vi "TraverseDoAllChannels.vi"(0 "Current Pulses positions for all channels":sgl[](array[numeric]), 1 "Current Pos In Eng units of all channels":sgl[](array[numeric]) format="%.2f", 2 "Counters Reset?":bool, 5 "Backlash Compensation?":bool, 7 "Home":T3, 9 "Mode":T4, 11 "Position Steps":sgl[][](array[numeric]) format="%.2f", 12 "Channel Properties":T1[](array[typedef]) {"Current Pos" format="%.2f"; "Backlash/Eng units" format="%.2f"; "Pulses/rev" format="%.2f"; "Pos Tolerance" format="%.2f"; "Pulses/unit" format="%.2f"; "Acc. Min" format="%.2f"; "Acc. Max" format="%.2f"; "Vel. Min" format="%.2f"; "Vel. Max" format="%.2f"; "Acc. Default" format="%.2f"; "Vel. Default" format="%.2f"}, 13 "Last Part of Move?":bool, 14 "Traverse Name":string="EnFlo Tunnel") -> (4 "Achieved Pos In Eng units of all channels":sgl[](array[numeric]) format="%.2f", 6 "Current Pulses positions for all channels Out":sgl[](array[numeric]), 8 "Moved?":bool, 10 "Error String":string, 15 "Channel Properties Out":T1[](array[typedef]) {"Current Pos" format="%.2f"; "Backlash/Eng units" format="%.2f"; "Pulses/rev" format="%.2f"; "Pos Tolerance" format="%.2f"; "Pulses/unit" format="%.2f"; "Acc. Min" format="%.2f"; "Acc. Max" format="%.2f"; "Vel. Min" format="%.2f"; "Vel. Max" format="%.2f"; "Acc. Default" format="%.2f"; "Vel. Default" format="%.2f"})   [LabVIEW 2022 SP3]
uses:
  Anemometry/Anemometry Sub Vis/Gen Trav/Trav_mode.ctl
  Anemometry/Anemometry Sub Vis/Controls/Home.ctl
  ~subVIs/DriveProperties.ctl
  ~subVIs/Traverse Type.ctl
  ~subVIs/DriveGotoCluster.ctl
  ~subVIs/DriveConfigGlobal.vi
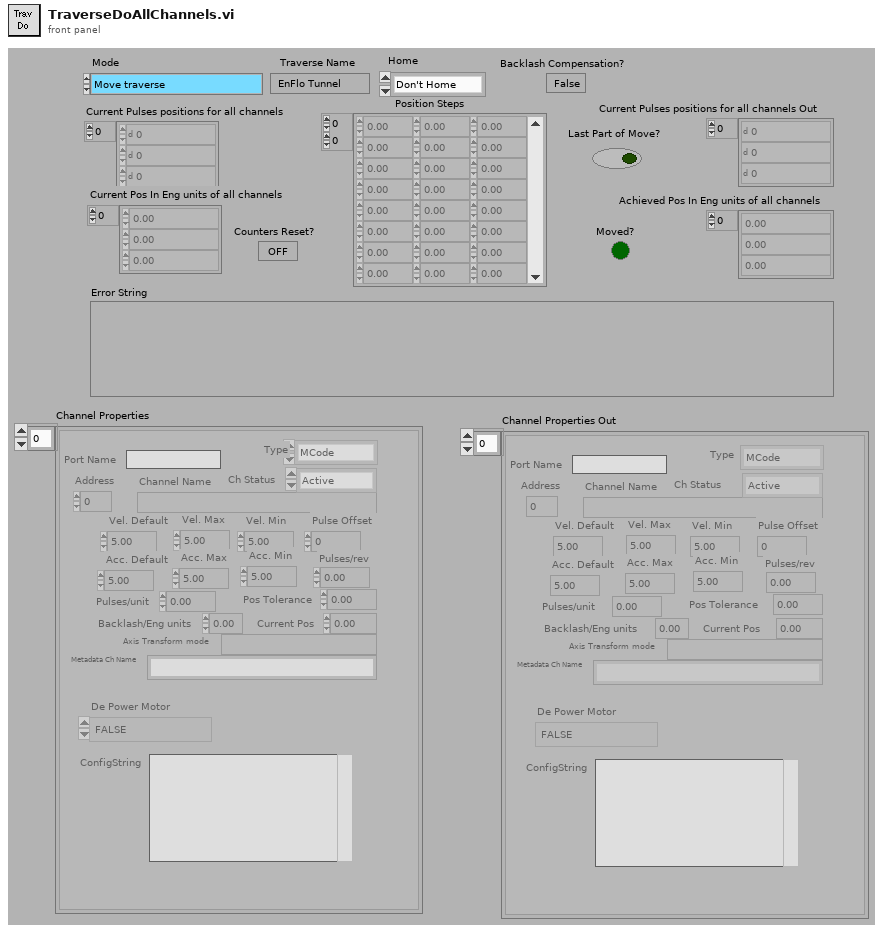
[diagram p1: front panel]
types:
  T1 = typedef "DriveProperties.ctl" = cluster{"Channel Name":string, "Vel. Default":sgl, "Acc. Default":sgl, "Vel. Max":sgl, "Vel. Min":sgl, "Acc. Max":sgl, "Acc. Min":sgl, "Pulses/unit":sgl, "Address":u8, "Pulse Offset":i32, "Pos Tolerance":sgl, "Pulses/rev":sgl, "Backlash/Eng units":sgl, "Current Pos":sgl, "Ch Status":enum16{"Active", "Offline", "Simulate"}, "Port Name":string, "Axis Transform mode":string, "Metadata Ch Name":string, "Type":T2, "De Power Motor":enum16{"TRUE", "FALSE"}, "ConfigString":string}
  T2 = typedef "Traverse Type.ctl" = enum16{"MCode", "Dynamixel"}
  T3 = typedef "Home.ctl" = enum16{"Don't Home", "Home  +X", "Home  -X", "Home  +Y", "Home  -Y", "Home  +Z", "Home  -Z"}
  T4 = typedef "Trav_mode.ctl" = enum16{"Move traverse", "Read traverse position", "Teach Position"}
  T5 = enum16{"Load setup from excel file", "Save setup to excel file"}
  T6 = typedef "DriveGotoCluster.ctl" = cluster{"Channel name":string, "Go To Position":dbl}
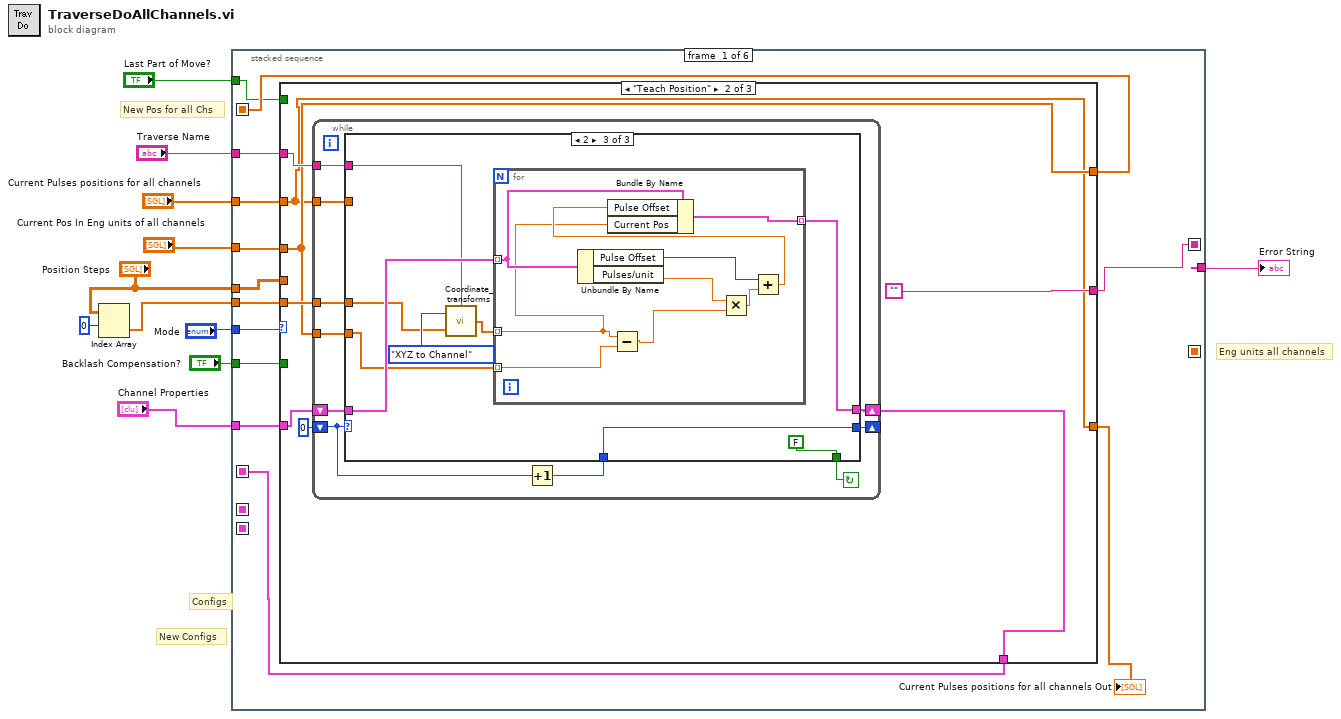
[diagram p0: block diagram]
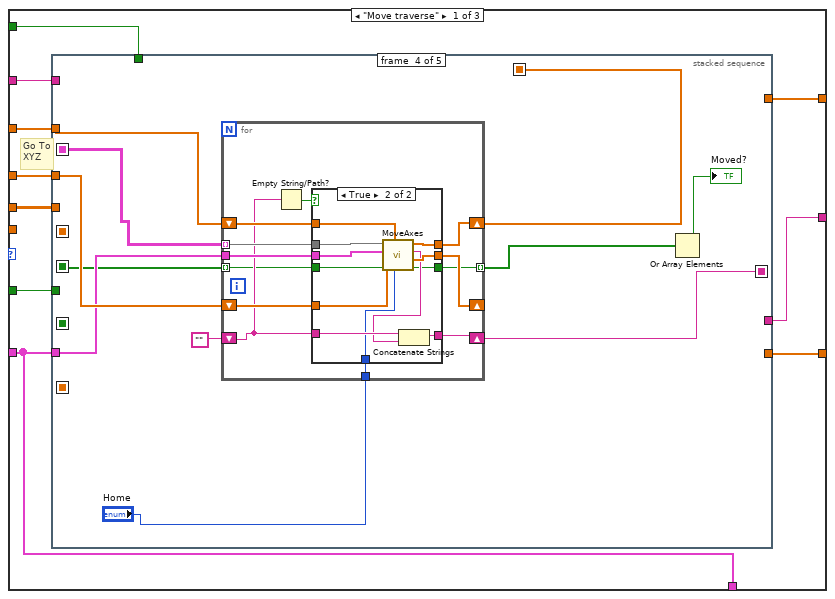
[diagram p2: hidden frame]
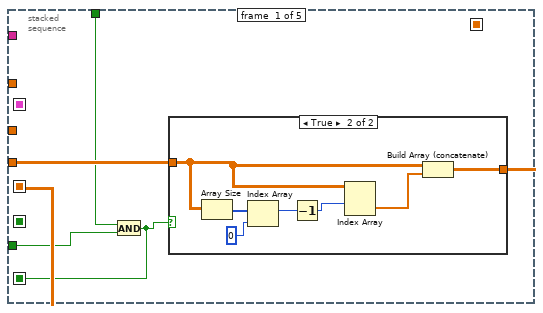
[diagram p3: hidden frame]
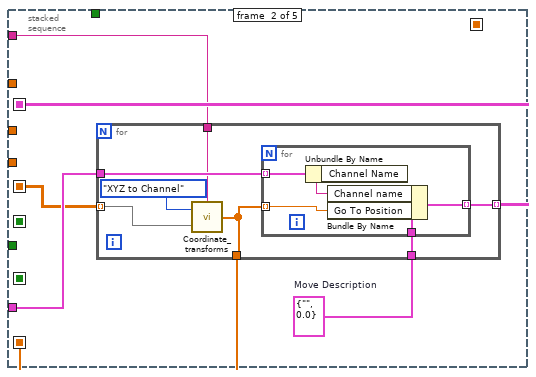
[diagram p5: hidden frame]
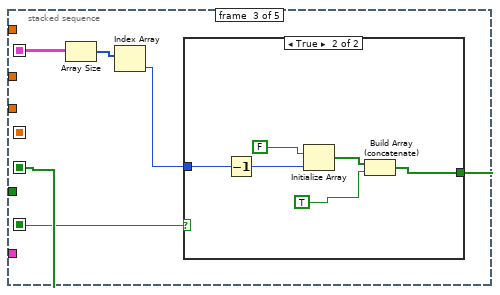
[diagram p6: hidden frame]
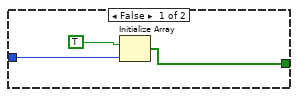
[diagram p7: hidden frame]
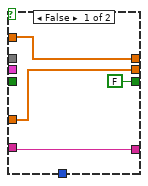
[diagram p8: hidden frame]
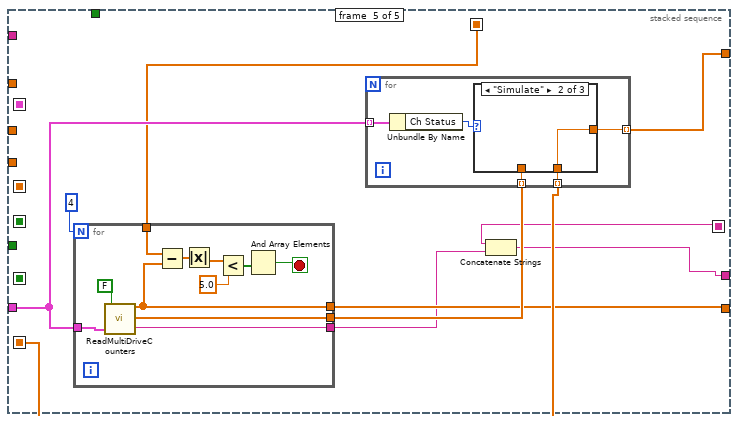
[diagram p9: hidden frame]
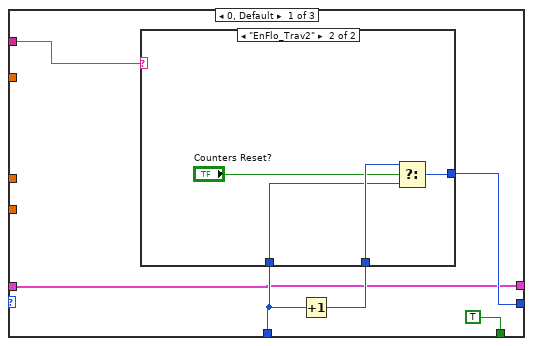
[diagram p12: hidden frame]
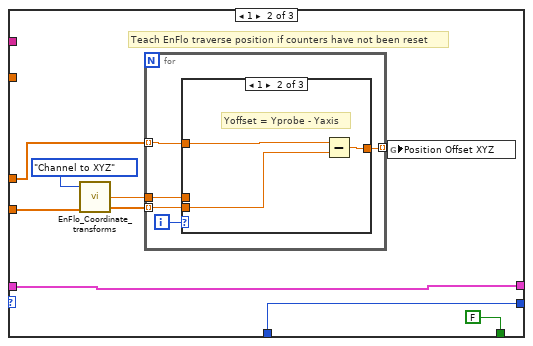
[diagram p14: hidden frame]
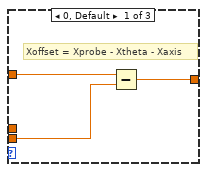
[diagram p15: hidden frame]
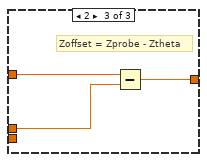
[diagram p16: hidden frame]
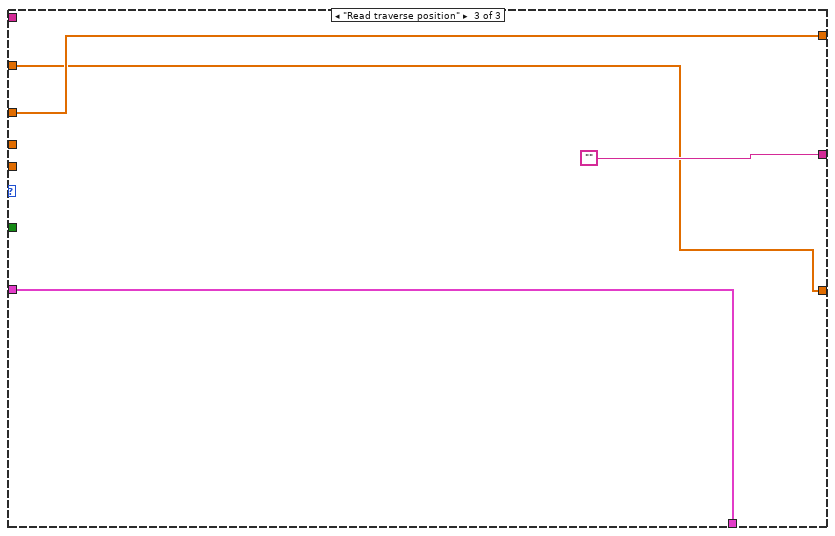
[diagram p17: hidden frame]
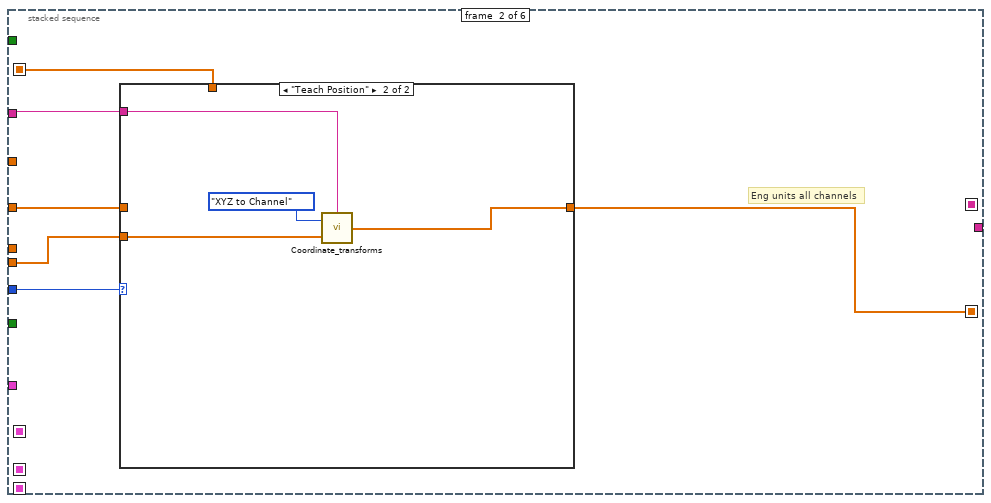
[diagram p18: hidden frame]
diagram:
  # "New Pos for all Chs"
  # "Eng units all channels"
  # "New Configs"
  # "Configs"
  n1 = Index Array(array="Position Steps", index (row)=0 ("Index")) -> (element=w3:sgl[])  [unwired: 1 in]
  n2 = stacked-sequence {
    seq-local: [_ w225 _ _ _ _] -> [_ _ _ w245 _ _]
    seq-local: [w23 _ _ _ _ _] -> [_ _ _ w247 _ _]
    seq-local: [_ _ _ w246 _ _] -> [_ _ _ _ w254 _]
    seq-local: [w15 _ _ _ _ _] -> [_ w222 _ _ _ _]
    seq-local: [_ _ _ _ w251 _] -> [_ _ _ _ _ w261]
    seq-local: [w12 _ _ _ _ _] -> [_ _ w235 _ _ _]
    tunnel: "Mode" -> [w24 w226 w233 _ _ w262]
    tunnel: "Current Pos In Eng units of all channels" -> [w21 w227 _ _ _ _]
    tunnel: "Channel Properties" -> [w22 _ _ _ _ _]
    tunnel: "Current Pulses positions for all channels" -> [w20 _ _ _ _ _]
    tunnel: [_ _ w234 _ _ _] -> w8
    tunnel: "Traverse Name" -> [w19 w224 _ _ w253 w260]
    tunnel: "Position Steps" -> [w18 _ _ _ _ _]
    tunnel: "Backlash Compensation?" -> [w17 _ _ _ _ _]
    tunnel: w3 -> [w16 w223 _ _ _ _]
    tunnel: "Last Part of Move?" -> [w13 _ w236 _ w252 _]
    frame #0 {
      n3 = case shown="\"Teach Position\"" w24 {
        tunnel: [w34 w152 w221] -> w23
        tunnel: w22 -> [w34 w153 w221]
        tunnel: w21 -> [w32 w149 w219]
        tunnel: w20 -> [w33 w148 w218]
        tunnel: [w31 "" ""] -> w12
        tunnel: w19 -> [w29 w154 _]
        tunnel: w18 -> [w30 _ _]
        tunnel: w17 -> [w28 _ _]
        tunnel: w16 -> [_ w150 _]
        tunnel: [w27 w149 w219] -> w15
        tunnel: [w26 w148 w218] -> w14
        tunnel: w13 -> [w25 _ _]
        frame "Move traverse" {
          # "Go To\nXYZ"
          n4 = stacked-sequence {
            seq-local: [_ w51 _ _ _] -> [_ _ w70 w87 _]
            seq-local: [w39 _ _ _ _] -> [_ w50 _ _ _]
            seq-local: [_ _ _ w85 _] -> [_ _ _ _ w123]
            seq-local: [_ w48 _ _ _] -> [_ _ _ _ w125]
            seq-local: [w35 _ _ _ _] -> [_ _ w66 _ _]
            seq-local: [_ _ w69 _ _] -> [_ _ _ w81 _]
            seq-local: [_ _ _ w80 _] -> [_ _ _ _ w120]
            tunnel: w34 -> [_ w52 _ w86 w128]
            tunnel: w33 -> [_ _ _ w90 _]
            tunnel: w32 -> [_ _ _ w89 _]
            tunnel: [_ _ _ _ w121] -> w31
            tunnel: w30 -> [w38 _ _ _ _]
            tunnel: w29 -> [_ w49 _ _ _]
            tunnel: w28 -> [w37 _ _ _ _]
            tunnel: [_ _ _ _ w127] -> w27
            tunnel: [_ _ _ _ w124] -> w26
            tunnel: w25 -> [w36 _ _ _ _]
            frame #0 {
              n5 = And(x=w36, y=w37) -> (x .and. y?=w35:bool)
              n6 = case shown="True" w35 {
                tunnel: w38 -> [w40 w42]
                tunnel: [w40 w41] -> w39
                frame False {
                }
                frame True {
                  n7 = Array Size(array=w42) -> (size(s)=w47:i32[])
                  n8 = Index Array(array=w47, index=0 ("Index")) -> (element=w45:i32)
                  n9 = Decrement(x=w45) -> (x-1=w44:i32)
                  n10 = Index Array(array=w42, index (row)=w44) -> (element=w43:sgl[])  [unwired: 1 in]
                  n11 = Build Array (concatenate)(w42, w43) -> (w41:sgl[][])
                }
              }
            }
            frame #1 {
              w53 = T6 {"Channel name"="", "Go To Position"=0.0}  # Move Description
              n12 = for {
                tunnel: w53 -> [w60]
                tunnel: w52 -> [w59]
                tunnel: [w58] -> w51 mode=indexing
                tunnel: w50 -> [w55] mode=indexing
                tunnel: w49 -> [w56]
                tunnel: [w54] -> w48
                n13 = call "Coordinate_transforms.vi"("Traverse Name"=w56, "Input"=w55, "Mode"=enum16{"XYZ to Channel", "Channel to XYZ"}."XYZ to Channel") -> ("Output"=w54:sgl[])
                n14 = for {
                  tunnel: w54 -> [w65] mode=indexing
                  tunnel: [w64] -> w58 mode=indexing
                  tunnel: w59 -> [w62] mode=indexing
                  tunnel: w60 -> [w61]
                  n15 = Unbundle By Name(w62) -> ("Channel Name"=w63:string)
                  n16 = Bundle By Name(cluster=w61, "Channel name"=w63, "Go To Position"=w65) -> (w64:T6)
                }
              }
            }
            frame #2 {
              n17 = Array Size(array=w70) -> (size(s)=w68:i32[])
              n18 = Index Array(array=w68) -> (element=w67:i32)  [unwired: 1 in]
              n19 = case shown="True" w66 {
                tunnel: [w71 w79] -> w69
                tunnel: w67 -> [w72 w77]
                frame False {
                  n20 = Initialize Array(TRUE, w72) -> (w71:bool[])
                }
                frame True {
                  n21 = Decrement(x=w77) -> (x-1=w78:i32)
                  n22 = Initialize Array(FALSE, w78) -> (w75:bool[])
                  n23 = Build Array (concatenate)(w75, TRUE) -> (w79:bool[])
                }
              }
            }
            frame #3 {
              n24 = for {
                tunnel: w87 -> [w102] mode=indexing
                tunnel: w86 -> [w101]
                shift-right: [w98] -> w80
                shift-left: w90 -> [w97]
                shift-right: [w99] -> _
                shift-left: w89 -> [w100]
                shift-right: [w96] -> w85
                shift-left: "" -> [w95]
                tunnel: "Home" -> [w93]
                tunnel: [w92] -> w83 mode=indexing
                tunnel: w81 -> [w91] mode=indexing
                n25 = Empty String/Path?(string/path=w95) -> (empty?=w94:bool)
                n26 = case shown="True" w94 {
                  tunnel: w102 -> [_ w118]
                  tunnel: w101 -> [_ w117]
                  tunnel: w100 -> [w105 w116]
                  tunnel: [w105 w115] -> w99
                  tunnel: [w106 w114] -> w98
                  tunnel: w97 -> [w106 w113]
                  tunnel: [w104 w110] -> w96
                  tunnel: w95 -> [w104 w112]
                  tunnel: w93 -> [_ w109]
                  tunnel: [FALSE ("Moved?") w108] -> w92
                  tunnel: w91 -> [_ w107]
                  frame False {
                  }
                  frame True {
                    n27 = call "MoveAxes.vi"("Home"=w109, "Current Pulses In"=w113, "Pos without backlash"=w107, "Current Pos In"=w116, "Channel Properties"=w117, "GoTo Array (Eng units all channels)"=w118) -> ("Moved?"=w108:bool, "Current Pos Out"=w115:dbl[], "Error String"=w111:string, "Current Pulses Out"=w114:dbl[])
                    n28 = Concatenate Strings(w112, w111) -> (w110:string)
                  }
                }
              }
              n29 = Or Array Elements(Boolean array=w83) -> (logical OR=→"Moved?":bool)
            }
            frame #4 {
              n30 = for {
                N: 4 -> [_]
                tunnel: w128 -> [w138]
                tunnel: [w137] -> w126
                tunnel: [w135] -> w124
                tunnel: [w136] -> w122
                tunnel: w120 -> [w134]
                stop <- w129 stop-if-true
                n31 = call "ReadMultiDriveCounters.vi"("Recheck if Moved?"=FALSE, "Channel Properties"=w138) -> ("Pulses"=w135:sgl[], "Eng units"=w137:sgl[], "Error String"=w136:string)  [unwired: 1 in, 1 out]
                n32 = Subtract(x=w134, y=w135) -> (x-y=w133:dbl[])
                n33 = Absolute Value(x=w133) -> (abs(x)=w132:dbl[])
                n34 = Less?(x=w132, y=5.0) -> (x < y?=w130:bool[])
                n35 = And Array Elements(Boolean array=w130) -> (logical AND=w129:bool)
              }
              n36 = for {
                tunnel: w128 -> [w144] mode=indexing
                tunnel: [w142] -> w127 mode=indexing
                tunnel: w126 -> [w141] mode=indexing
                tunnel: w125 -> [w140] mode=indexing
                n37 = Unbundle By Name(w144) -> ("Ch Status"=w143:enum16{"Active", "Offline", "Simulate"})
                n38 = case shown="\"Simulate\"" w143 {
                  tunnel: [w145 w146 w147] -> w142
                  tunnel: w141 -> [w145 _ w147]
                  tunnel: w140 -> [_ w146 _]
                  frame "Active" {
                  }
                  frame "Simulate" {
                  }
                  frame "Offline" {
                  }
                }
              }
              n39 = Concatenate Strings(w123, w122) -> (w121:string)
            }
          }
        }
        frame "Teach Position" {
          n40 = while {
            tunnel: w150 -> [w156]
            shift-left: w153 -> [w158]
            shift-right: [w157] -> w152
            tunnel: w149 -> [w159]
            tunnel: w148 -> [w160]
            tunnel: w154 -> [w161]
            shift-left: 0 -> [w165]
            shift-right: [w162] -> _
            stop <- w164 continue-if-true
            n41 = Increment(x=w165) -> (x+1=w163:i32)
            n42 = case shown="2" w165 {
              tunnel: [TRUE FALSE FALSE] -> w164
              tunnel: w163 -> [w168 w179 w208]
              tunnel: [w169 w179 w208] -> w162
              tunnel: w161 -> [w170 _ w201]
              tunnel: w160 -> [_ _ _]
              tunnel: w159 -> [_ w180 w202]
              tunnel: w158 -> [w166 w178 w206]
              tunnel: [w166 w178 w205] -> w157
              tunnel: w156 -> [_ w177 w200]
              frame 0, Default {
                n43 = Increment(x=w168) -> (x+1=w167:i32)
                n44 = case shown="\"EnFlo_Trav2\"" w170 {
                  tunnel: [w172 w176] -> w169
                  tunnel: w168 -> [_ w174]
                  tunnel: w167 -> [w172 w175]
                  frame "A_Tunnel", Default {
                  }
                  frame "EnFlo_Trav2" {
                    n45 = Select(t=w175, s="Counters Reset?", f=w174) -> (s? t:f=w176:i32)
                  }
                }
              }
              frame 1 {
                # "Teach EnFlo traverse position if counters have not been reset"
                n46 = call "EnFlo_Coordinate_transforms.vi"("Input"=w180, "Mode"=enum16{"XYZ to Channel", "Channel to XYZ"}."Channel to XYZ") -> ("Output"=w183:dbl[], "Z theta"=w182:dbl)  [unwired: 2 out]
                n47 = for {
                  tunnel: w177 -> [w189] mode=indexing
                  tunnel: w183 -> [w188] mode=indexing
                  tunnel: [w187] -> w184 mode=indexing
                  tunnel: w182 -> [w186]
                  i -> [w190]
                  n48 = case shown="1" w190 {
                    tunnel: w189 -> [w193 w196 w199]
                    tunnel: w188 -> [w192 w195 _]
                    tunnel: [w191 w194 w197] -> w187
                    tunnel: w186 -> [_ _ w198]
                    frame 0, Default {
                      # "Xoffset = Xprobe - Xtheta - Xaxis"
                      n49 = Subtract(x=w193, y=w192) -> (x-y=w191:dbl)
                    }
                    frame 1 {
                      # "Yoffset = Yprobe - Yaxis"
                      n50 = Subtract(x=w196, y=w195) -> (x-y=w194:dbl)
                    }
                    frame 2 {
                      # "Zoffset = Zprobe - Ztheta"
                      n51 = Subtract(x=w199, y=w198) -> (x-y=w197:dbl)
                    }
                  }
                }
                n52 = global write "DriveConfigGlobal.vi" "Position Offset XYZ"(w184) -> ()
              }
              frame 2 {
                n53 = call "Coordinate_transforms.vi"("Traverse Name"=w201, "Input"=w200, "Mode"=enum16{"XYZ to Channel", "Channel to XYZ"}."XYZ to Channel") -> ("Output"=w203:sgl[])
                n54 = for {
                  tunnel: w206 -> [w217] mode=indexing
                  tunnel: [w215] -> w205 mode=indexing
                  tunnel: w202 -> [w213] mode=indexing
                  tunnel: w203 -> [w209] mode=indexing
                  n55 = Unbundle By Name(w217) -> ("Pulse Offset"=w214:i32, "Pulses/unit"=w212:sgl)
                  n56 = Subtract(x=w209, y=w213) -> (x-y=w210:sgl)
                  n57 = Multiply(x=w212, y=w210) -> (x*y=w211:sgl)
                  n58 = Add(x=w214, y=w211) -> (x+y=w216:sgl)
                  n59 = Bundle By Name(cluster=w217, "Pulse Offset"=w216, "Current Pos"=w209) -> (w215:T1)
                }
              }
            }
          }
        }
        frame "Read traverse position" {
        }
      }
      "Current Pulses positions for all channels Out" <- w14
    }
    frame #1 {
      # "Eng units all channels"
      n60 = case shown="\"Teach Position\"" w226 {
        tunnel: w227 -> [_ _]
        tunnel: [w228 w231] -> w225
        tunnel: w224 -> [_ w230]
        tunnel: w223 -> [_ w229]
        tunnel: w222 -> [w228 _]
        frame "Move traverse", Default {
        }
        frame "Teach Position" {
          n61 = call "Coordinate_transforms.vi"("Traverse Name"=w230, "Input"=w229, "Mode"=enum16{"XYZ to Channel", "Channel to XYZ"}."XYZ to Channel") -> ("Output"=w231:sgl[])
        }
      }
    }
    frame #2 {
      n62 = case shown="Default" w233 {
        tunnel: w236 -> [w239 _]
        tunnel: w235 -> [w238 w244]
        tunnel: [w237 w244] -> w234
        frame "Move traverse" {
          n63 = case shown="True" w239 {
            tunnel: w238 -> [w240 w242]
            tunnel: [w240 w241] -> w237
            frame False {
            }
            frame True {
              n64 = call "Shut_down_all_Axis.vi"() -> ("Error String"=w243:string)  [unwired: 1 in]
              n65 = Concatenate Strings(w242, w243) -> (w241:string)
            }
          }
        }
        frame Default {
        }
      }
    }
    frame #3 {
      n66 = for {
        tunnel: [w250] -> w246 mode=indexing
        tunnel: w247 -> [w249] mode=indexing
        tunnel: w245 -> [w248] mode=indexing
        n67 = Bundle By Name(cluster=w249, "Current Pos"=w248) -> (w250:T1)
      }
      "Achieved Pos In Eng units of all channels" <- w245
    }
    frame #4 {
      n68 = case shown="True" w252 {
        tunnel: w254 -> [w255 w258]
        tunnel: w253 -> [_ w257]
        tunnel: [w255 w256] -> w251
        frame False {
        }
        frame True {
          n69 = call "Read_Write_Trav_position.vi"("Channel Properties"=w258, "Mode"=T5."Save setup to excel file", "Traverse Name"=w257) -> ("Channel Properties Out"=w256:T1[])  [unwired: 1 out]
        }
      }
      "Channel Properties Out" <- w251
    }
    frame #5 {
      n70 = case shown="\"Move traverse\", Default" w262 {
        tunnel: w261 -> [_ w264]
        tunnel: w260 -> [_ w263]
        frame "Move traverse", Default {
        }
        frame "Teach Position" {
          n71 = stacked-sequence {
            tunnel: w264 -> [w267 _]
            tunnel: w263 -> [_ w277]
            frame #0 {
              n72 = global read "DriveConfigGlobal.vi" "Channel Properties"() -> (w266:T1[])
              n73 = for {
                tunnel: w266 -> [w276] mode=indexing
                tunnel: [w275] -> w268 mode=indexing
                n74 = Unbundle By Name(w276) -> ("Channel Name"=w275:string)
              }
              n75 = for {
                tunnel: w268 -> [w274]
                tunnel: w267 -> [w269] mode=indexing
                shift-right: [w271] -> w265
                shift-left: w266 -> [w272]
                n76 = Unbundle By Name(w269) -> ("Channel Name"=w273:string)
                n77 = Search 1D Array(1D array=w274, element=w273) -> (index of element=w270:i32)  [unwired: 1 out]
                n78 = Replace Array Subset(array=w272, new element=w269, index=w270) -> (w271:T1[])
              }
              n79 = global write "DriveConfigGlobal.vi" "Channel Properties"(w265) -> ()
            }
            frame #1 {
              n80 = call "Read_Write_Trav_Config.vi"("Traverse Name"=w277, "Mode"=T5."Save setup to excel file") -> ()  [unwired: 1 out]
            }
          }
        }
      }
    }
  }
  "Error String" <- w8
